vi "Get Next Value.vi"(11 "Value In":i64[](array[numeric])) -> (3 "Value Out":i64[](array[numeric]))   [LabVIEW 2021]
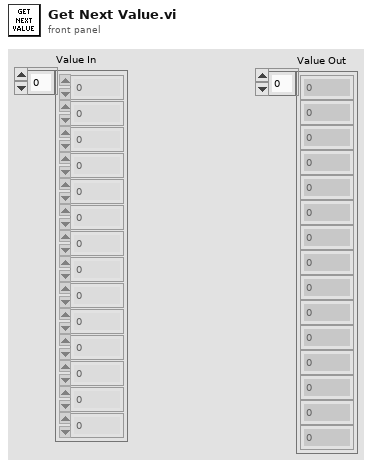
[diagram p1: front panel]
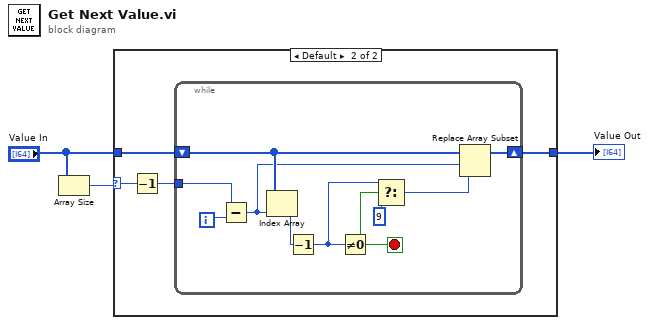
[diagram p0: block diagram]
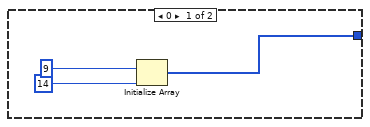
[diagram p2: hidden frame]
diagram:
  n1 = Array Size(array="Value In") -> (size(s)=w3:i32)
  n2 = case shown="Default" w3 {
    selector: w3 -> [_ w8]
    tunnel: "Value In" -> [_ w10]
    tunnel: [w4 w9] -> w1
    frame 0 {
      n3 = Initialize Array(i64 9 ("element"), 14 ("dimension size")) -> (w4:i64[])
    }
    frame Default {
      n4 = Decrement(x=w8) -> (x-1=w7:i32)
      n5 = while {
        shift-right: [w12] -> w9
        shift-left: w10 -> [w19]
        tunnel: w7 -> [w11]
        i -> [w20]
        stop <- w17 stop-if-true
        n6 = Subtract(x=w11, y=w20) -> (x-y=w18:i32)
        n7 = Index Array(array=w19, index=w18) -> (element=w15:i64)
        n8 = Decrement(x=w15) -> (x-1=w16:i64)
        n9 = Not Equal To 0?(x=w16) -> (x != 0?=w17:bool)
        n10 = Select(t=w16, s=w17, f=i64 9) -> (s? t:f=w13:i64)
        n11 = Replace Array Subset(array=w19, new element=w13, index=w18) -> (w12:i64[])
      }
    }
  }
  "Value Out" <- w1
